vi "ExposeGetCSComNPMessageInfo.vi"(11 "NPMessage":refnum<k24>) -> (3 "MessageInfo":T1 {"Message Type" items=["Error"=1, "Warning"=2, "Create"=4, "Destroy"=8, "Invoke"=16, "Get"=32, "Set"=64, "Response"=128]})   [LabVIEW 2017]
uses:
  C:/Code/CMCryoSysCode/Expose/COM/CSCom/CSCom/bin/Release/CSCom.dll
  COM/CSCom/CSCom/bin/Release/CSCom.dll
  ExposeMessage.ctl
  Events/ExposeMessageType.ctl
  Mapper/ExposeObjectMapNamepathData.ctl
  Mapper/ExposeMapperDataTypeEnum.ctl
  Mapper/ExposeObjectMapContainerTypeEnum.ctl
panel:
  out "String rep":string
  out "NumericMessageType":i32
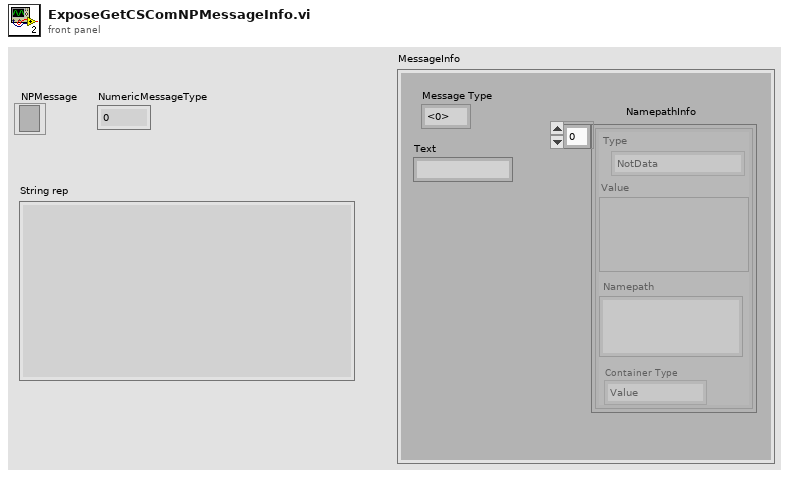
[diagram p1: front panel]
types:
  T1 = typedef "ExposeMessage.ctl" = cluster{"Message Type":T2, "Text":string, "NamepathInfo":T3[]}
  T2 = typedef "ExposeMessageType.ctl" = i32
  T3 = typedef "ExposeObjectMapNamepathData.ctl" = cluster{"Type":T4, "Value":variant, "Namepath":string, "Container Type":T5}
  T4 = typedef "ExposeMapperDataTypeEnum.ctl" = enum16{"NotData", "int8", "byte", "int16", "uint16", "int32", "uint32", "int64", "uint64", "Single", "Double", "String", "Boolean", "Container"}
  T5 = typedef "ExposeObjectMapContainerTypeEnum.ctl" = enum16{"Value", "Array", "Waveform", "NetContainer"}
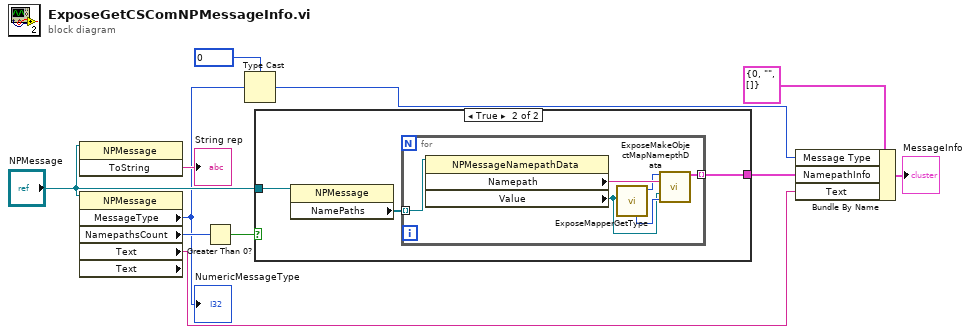
[diagram p0: block diagram]
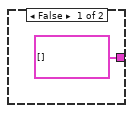
[diagram p2: hidden frame]
diagram:
  w8 = T2 0 items=["Error"=1, "Warning"=2, "Create"=4, "Destroy"=8, "Invoke"=16, "Get"=32, "Set"=64, "Response"=128] ("Message Type")
  n1 = invoke class="NPMessage" method="ToString"(reference="NPMessage") -> ("ToString"=→"String rep":string)  [unwired: 2 in, 2 out]
  n2 = property class="NPMessage" props=["MessageType", "NamepathsCount", "Text", "Text"](reference="NPMessage") -> ("MessageType"=w2:i32, "NamepathsCount"=w3:i32, "Text"=w4:string)  [unwired: 1 in, 3 out]
  "NumericMessageType" <- w2
  n3 = Greater Than 0?(x=w3) -> (x > 0?=w11:bool)
  n4 = Type Cast(type=w8, x=w2) -> (*(type *) &x=w7:T2)
  n5 = case shown="True" w11 {
    tunnel: "NPMessage" -> [_ w15]
    tunnel: [T3[] [] w13] -> w1
    frame False {
    }
    frame True {
      n6 = property class="NPMessage"(reference=w15) -> ("NamePaths"=w14:refnum<k24>[])  [unwired: 1 in, 2 out]
      n7 = for {
        tunnel: w14 -> [w17] mode=indexing
        tunnel: [w18] -> w13 mode=indexing
        n8 = property class="NPMessageNamepathData"(reference=w17) -> ("Namepath"=w21:string, "Value"=w16:refnum<k24>)  [unwired: 1 in, 2 out]
        n9 = call "ExposeMapperGetType.vi"("Value"=w16) -> ("DataType"=w20:T4, "Container Type (Labview Value type)"=w19:T5)  [unwired: 5 in, 4 out]
        n10 = call "ExposeMakeObjectMapNamepthData.vi"("ObjectMapType"=w20, "namepath"=w21, "value"=w16, "Labview Contriner type"=w19) -> ("MatlabDataBundle"=w18:T3)  [unwired: 11 in]
      }
    }
  }
  n11 = Bundle By Name(cluster=T1 {"Message Type"=0, "Text"="", "NamepathInfo"=[]} ("MessageInfo"), "Message Type"=w7, "NamepathInfo"=w1, "Text"=w4) -> (→"MessageInfo":T1)
